vi "输入数据解析.vi"(0 "单个参数补充":dbl, 1 "从板号":dbl=1.0, 2 "主板二维码":string="BNET01", 3 "从板二维码":string="BNET01", 5 "主板引用":refnum<vi>, 7 "从板引用":refnum<vi>, 9 "主板选项":string="三级故障阀值", 11 "枚举":enum16{"主板", "从板"}(ring), 12 "快换":bool caption="快换写入") -> (4 "输出数组":dbl[][](array[numeric]), 6 "数组长度":dbl[](array[numeric]), 8 "循环次数":i32, 10 "命令":u32, 14 "名称":string[](array[string]), 15 "命令序号":u32[](array[numeric]))   [LabVIEW 2013] (continued)
                    n6601 = call "输入分辨率计算-EV05.vi"("1字节?"=FALSE, "数值"=w16862, "分辨率"=0.001) -> ("低字节"=w16864:dbl, "高字节1"=w16865:dbl)  [unwired: 2 in, 5 out]
                  }
                  frame Disabled {
                    w16868 = 255 ("高字节1")
                  }
                }
                n6602 = Build Array(w16861, w16860) -> (w16859:dbl[])
              }
              frame 1 {
                # "电压过低"
                n6603 = disable-structure shown="启用" {
                  disable-tunnel: [w16876 w16879] -> w16872
                  disable-tunnel: [w16875 w16879] -> w16871
                  disable-tunnel: w16869 -> [w16874 _]
                  frame Disabled {
                    n6604 = Unbundle By Name(w16874) -> ("电压过低"=w16873:dbl)
                    n6605 = call "输入分辨率计算-EV05.vi"("1字节?"=FALSE, "数值"=w16873, "分辨率"=0.1) -> ("低字节"=w16875:dbl, "高字节1"=w16876:dbl)  [unwired: 2 in, 5 out]
                  }
                  frame Enabled {
                    w16879 = 255 ("高字节1")
                  }
                }
                n6606 = Build Array(w16872, w16871) -> (w16870:i32[])
              }
              frame 2 {
                # "电压不均衡"
                n6607 = disable-structure shown="启用" {
                  disable-tunnel: [w16887 w16890] -> w16883
                  disable-tunnel: [w16886 w16890] -> w16882
                  disable-tunnel: w16880 -> [w16885 _]
                  frame Disabled {
                    n6608 = Unbundle By Name(w16885) -> ("电压不均衡(V)"=w16884:dbl)
                    n6609 = call "输入分辨率计算-EV05.vi"("1字节?"=FALSE, "数值"=w16884, "分辨率"=0.1) -> ("低字节"=w16886:dbl, "高字节1"=w16887:dbl)  [unwired: 2 in, 5 out]
                  }
                  frame Enabled {
                    w16890 = 255 ("高字节1")
                  }
                }
                n6610 = Build Array(w16883, w16882) -> (w16881:i32[])
              }
              frame 3 {
                # "温度过高"
                n6611 = disable-structure shown="启用" {
                  disable-tunnel: [w16897 255 ("高字节1")] -> w16893
                  disable-tunnel: w16891 -> [w16895 _]
                  frame Disabled {
                    n6612 = Unbundle By Name(w16895) -> ("温度过高"=w16894:dbl)
                    n6613 = call "输入分辨率计算-EV05.vi"("1字节?"=TRUE, "数值"=w16894, "偏移量"=-40.0, "分辨率"=1.0) -> ("高字节1"=w16897:dbl)  [unwired: 1 in, 6 out]
                  }
                  frame Enabled {
                  }
                }
                n6614 = Build Array(w16893) -> (w16892:i32[])
              }
              frame 4 {
                # "温度过低"
                n6615 = disable-structure shown="启用" {
                  disable-tunnel: [w16907 255 ("高字节1")] -> w16903
                  disable-tunnel: w16901 -> [w16905 _]
                  frame Disabled {
                    n6616 = Unbundle By Name(w16905) -> ("温度过低"=w16904:dbl)
                    n6617 = call "输入分辨率计算-EV05.vi"("1字节?"=TRUE, "数值"=w16904, "偏移量"=-40.0, "分辨率"=1.0) -> ("高字节1"=w16907:dbl)  [unwired: 1 in, 6 out]
                  }
                  frame Enabled {
                  }
                }
                n6618 = Build Array(w16903) -> (w16902:i32[])
              }
              frame 5 {
                # "温度不均衡"
                n6619 = disable-structure shown="启用" {
                  disable-tunnel: [w16916 255 ("高字节1")] -> w16913
                  disable-tunnel: w16911 -> [w16915 _]
                  frame Disabled {
                    n6620 = Unbundle By Name(w16915) -> ("温度不均衡"=w16914:dbl)
                    n6621 = call "输入分辨率计算-EV05.vi"("1字节?"=TRUE, "数值"=w16914, "分辨率"=1.0) -> ("高字节1"=w16916:dbl)  [unwired: 2 in, 6 out]
                  }
                  frame Enabled {
                  }
                }
                n6622 = Build Array(w16913) -> (w16912:i32[])
              }
              frame 6 {
                # "SOC过低"
                n6623 = disable-structure shown="启用" {
                  disable-tunnel: w16922 -> [w16939 _]
                  disable-tunnel: [w16925 w16942] -> w16921
                  disable-tunnel: [w16924 w16942] -> w16920
                  frame Disabled {
                    n6624 = Unbundle By Name(w16939) -> ("SOC过低"=w16938:dbl)
                    n6625 = call "输入分辨率计算-EV05.vi"("1字节?"=FALSE, "数值"=w16938, "分辨率"=0.1) -> ("低字节"=w16927:dbl, "高字节1"=w16928:dbl)  [unwired: 2 in, 5 out]
                    n6626 = call "二进制解析-8.6.vi"("索引"=4, "数值"=0) -> ("低位子数组"=w16931:i32[])  [unwired: 3 out]
                    n6627 = call "二进制解析-8.6.vi"("索引"=4, "数值"=w16928) -> ("低位子数组"=w16934:i32[])  [unwired: 3 out]
                    n6628 = call "二进制解析-8.6.vi"("索引"=4, "数值"=w16927) -> ("低位子数组"=w16932:i32[], "高位子数组"=w16933:i32[])  [unwired: 2 out]
                    n6629 = Insert Into Array(array=w16934, new element=w16933) -> (w16936:i32[])  [unwired: 1 in]
                    n6630 = Insert Into Array(array=w16932, new element=w16931) -> (w16930:i32[])  [unwired: 1 in]
                    n6631 = call "数值二进制转十进制-8.6.vi"("子数组"=w16930) -> ("十进制数值"=w16925:i32)  [unwired: 4 out]
                    n6632 = call "数值二进制转十进制-8.6.vi"("子数组"=w16936) -> ("十进制数值"=w16924:i32)  [unwired: 4 out]
                  }
                  frame Enabled {
                    w16942 = 255 ("高字节1")
                  }
                }
                n6633 = Build Array(w16920, w16921) -> (w16923:i32[])
              }
            }
            n6634 = Insert Into Array(array=w16854, new element=w16853) -> (w16855:dbl[])  [unwired: 1 in]
          }
          n6635 = Build Array(w16848) -> (w16847:dbl[][])
        }
        frame "电压过低" {
          n6636 = Unbundle By Name(w16947) -> ("一级故障(从板)"=w16948:refnum<vi>)
          n6637 = property class="Clust (严格)"(reference=w16948) -> ("Value"=w16946:T8)  [unwired: 1 in, 2 out]
          n6638 = for {
            N: 7 -> [_]
            tunnel: w16946 -> [w16958]
            shift-right: [w16957] -> w16950
            shift-left: dbl[] [] -> [w16956]
            i -> [w16959]
            n6639 = case shown="1" w16959 {
              tunnel: w16958 -> [w16960 w16971 w16982 w16993 w17003 w17013 w17024]
              tunnel: [w16961 w16972 w16983 w16994 w17004 w17014 w17025] -> w16955
              frame 0, Default {
                # "电压过高"
                n6640 = disable-structure shown="启用" {
                  disable-tunnel: [w16967 w16970] -> w16963
                  disable-tunnel: [w16966 w16970] -> w16962
                  disable-tunnel: w16960 -> [w16965 _]
                  frame Disabled {
                    n6641 = Unbundle By Name(w16965) -> ("电压过高"=w16964:dbl)
                    n6642 = call "输入分辨率计算-EV05.vi"("1字节?"=FALSE, "数值"=w16964, "分辨率"=0.1) -> ("低字节"=w16966:dbl, "高字节1"=w16967:dbl)  [unwired: 2 in, 5 out]
                  }
                  frame Enabled {
                    w16970 = 255 ("高字节1")
                  }
                }
                n6643 = Build Array(w16963, w16962) -> (w16961:i32[])
              }
              frame 1 {
                # "电压过低"
                n6644 = disable-structure shown="启用" {
                  disable-tunnel: [w16978 w16981] -> w16974
                  disable-tunnel: [w16977 w16981] -> w16973
                  disable-tunnel: w16971 -> [w16976 _]
                  frame Enabled {
                    n6645 = Unbundle By Name(w16976) -> ("电压过低"=w16975:dbl)
                    n6646 = call "输入分辨率计算-EV05.vi"("1字节?"=FALSE, "数值"=w16975, "分辨率"=0.001) -> ("低字节"=w16977:dbl, "高字节1"=w16978:dbl)  [unwired: 2 in, 5 out]
                  }
                  frame Disabled {
                    w16981 = 255 ("高字节1")
                  }
                }
                n6647 = Build Array(w16974, w16973) -> (w16972:dbl[])
              }
              frame 2 {
                # "电压不均衡"
                n6648 = disable-structure shown="启用" {
                  disable-tunnel: [w16989 w16992] -> w16985
                  disable-tunnel: [w16988 w16992] -> w16984
                  disable-tunnel: w16982 -> [w16987 _]
                  frame Disabled {
                    n6649 = Unbundle By Name(w16987) -> ("电压不均衡(V)"=w16986:dbl)
                    n6650 = call "输入分辨率计算-EV05.vi"("1字节?"=FALSE, "数值"=w16986, "分辨率"=0.1) -> ("低字节"=w16988:dbl, "高字节1"=w16989:dbl)  [unwired: 2 in, 5 out]
                  }
                  frame Enabled {
                    w16992 = 255 ("高字节1")
                  }
                }
                n6651 = Build Array(w16985, w16984) -> (w16983:i32[])
              }
              frame 3 {
                # "温度过高"
                n6652 = disable-structure shown="启用" {
                  disable-tunnel: [w16999 255 ("高字节1")] -> w16995
                  disable-tunnel: w16993 -> [w16997 _]
                  frame Disabled {
                    n6653 = Unbundle By Name(w16997) -> ("温度过高"=w16996:dbl)
                    n6654 = call "输入分辨率计算-EV05.vi"("1字节?"=TRUE, "数值"=w16996, "偏移量"=-40.0, "分辨率"=1.0) -> ("高字节1"=w16999:dbl)  [unwired: 1 in, 6 out]
                  }
                  frame Enabled {
                  }
                }
                n6655 = Build Array(w16995) -> (w16994:i32[])
              }
              frame 4 {
                # "温度过低"
                n6656 = disable-structure shown="启用" {
                  disable-tunnel: [w17009 255 ("高字节1")] -> w17005
                  disable-tunnel: w17003 -> [w17007 _]
                  frame Disabled {
                    n6657 = Unbundle By Name(w17007) -> ("温度过低"=w17006:dbl)
                    n6658 = call "输入分辨率计算-EV05.vi"("1字节?"=TRUE, "数值"=w17006, "偏移量"=-40.0, "分辨率"=1.0) -> ("高字节1"=w17009:dbl)  [unwired: 1 in, 6 out]
                  }
                  frame Enabled {
                  }
                }
                n6659 = Build Array(w17005) -> (w17004:i32[])
              }
              frame 5 {
                # "温度不均衡"
                n6660 = disable-structure shown="启用" {
                  disable-tunnel: [w17018 255 ("高字节1")] -> w17015
                  disable-tunnel: w17013 -> [w17017 _]
                  frame Disabled {
                    n6661 = Unbundle By Name(w17017) -> ("温度不均衡"=w17016:dbl)
                    n6662 = call "输入分辨率计算-EV05.vi"("1字节?"=TRUE, "数值"=w17016, "分辨率"=1.0) -> ("高字节1"=w17018:dbl)  [unwired: 2 in, 6 out]
                  }
                  frame Enabled {
                  }
                }
                n6663 = Build Array(w17015) -> (w17014:i32[])
              }
              frame 6 {
                # "SOC过低"
                n6664 = disable-structure shown="启用" {
                  disable-tunnel: w17024 -> [w17041 _]
                  disable-tunnel: [w17027 w17044] -> w17023
                  disable-tunnel: [w17026 w17044] -> w17022
                  frame Disabled {
                    n6665 = Unbundle By Name(w17041) -> ("SOC过低"=w17040:dbl)
                    n6666 = call "输入分辨率计算-EV05.vi"("1字节?"=FALSE, "数值"=w17040, "分辨率"=0.1) -> ("低字节"=w17029:dbl, "高字节1"=w17030:dbl)  [unwired: 2 in, 5 out]
                    n6667 = call "二进制解析-8.6.vi"("索引"=4, "数值"=0) -> ("低位子数组"=w17033:i32[])  [unwired: 3 out]
                    n6668 = call "二进制解析-8.6.vi"("索引"=4, "数值"=w17030) -> ("低位子数组"=w17036:i32[])  [unwired: 3 out]
                    n6669 = call "二进制解析-8.6.vi"("索引"=4, "数值"=w17029) -> ("低位子数组"=w17034:i32[], "高位子数组"=w17035:i32[])  [unwired: 2 out]
                    n6670 = Insert Into Array(array=w17036, new element=w17035) -> (w17038:i32[])  [unwired: 1 in]
                    n6671 = Insert Into Array(array=w17034, new element=w17033) -> (w17032:i32[])  [unwired: 1 in]
                    n6672 = call "数值二进制转十进制-8.6.vi"("子数组"=w17032) -> ("十进制数值"=w17027:i32)  [unwired: 4 out]
                    n6673 = call "数值二进制转十进制-8.6.vi"("子数组"=w17038) -> ("十进制数值"=w17026:i32)  [unwired: 4 out]
                  }
                  frame Enabled {
                    w17044 = 255 ("高字节1")
                  }
                }
                n6674 = Build Array(w17022, w17023) -> (w17025:i32[])
              }
            }
            n6675 = Insert Into Array(array=w16956, new element=w16955) -> (w16957:dbl[])  [unwired: 1 in]
          }
          n6676 = Build Array(w16950) -> (w16949:dbl[][])
        }
        frame "电压过低(2)" {
          n6677 = Unbundle By Name(w17049) -> ("二级故障(从板)"=w17050:refnum<vi>)
          n6678 = property class="Clust (严格)"(reference=w17050) -> ("Value"=w17048:T8)  [unwired: 1 in, 2 out]
          n6679 = for {
            N: 7 -> [_]
            tunnel: w17048 -> [w17060]
            shift-right: [w17059] -> w17052
            shift-left: dbl[] [] -> [w17058]
            i -> [w17061]
            n6680 = case shown="1" w17061 {
              tunnel: w17060 -> [w17062 w17073 w17084 w17095 w17105 w17115 w17126]
              tunnel: [w17063 w17074 w17085 w17096 w17106 w17116 w17127] -> w17057
              frame 0, Default {
                # "电压过高"
                n6681 = disable-structure shown="启用" {
                  disable-tunnel: [w17069 w17072] -> w17065
                  disable-tunnel: [w17068 w17072] -> w17064
                  disable-tunnel: w17062 -> [w17067 _]
                  frame Disabled {
                    n6682 = Unbundle By Name(w17067) -> ("电压过高"=w17066:dbl)
                    n6683 = call "输入分辨率计算-EV05.vi"("1字节?"=FALSE, "数值"=w17066, "分辨率"=0.1) -> ("低字节"=w17068:dbl, "高字节1"=w17069:dbl)  [unwired: 2 in, 5 out]
                  }
                  frame Enabled {
                    w17072 = 255 ("高字节1")
                  }
                }
                n6684 = Build Array(w17065, w17064) -> (w17063:i32[])
              }
              frame 1 {
                # "电压过低"
                n6685 = disable-structure shown="启用" {
                  disable-tunnel: [w17080 w17083] -> w17076
                  disable-tunnel: [w17079 w17083] -> w17075
                  disable-tunnel: w17073 -> [w17078 _]
                  frame Enabled {
                    n6686 = Unbundle By Name(w17078) -> ("电压过低"=w17077:dbl)
                    n6687 = call "输入分辨率计算-EV05.vi"("1字节?"=FALSE, "数值"=w17077, "分辨率"=0.001) -> ("低字节"=w17079:dbl, "高字节1"=w17080:dbl)  [unwired: 2 in, 5 out]
                  }
                  frame Disabled {
                    w17083 = 255 ("高字节1")
                  }
                }
                n6688 = Build Array(w17076, w17075) -> (w17074:dbl[])
              }
              frame 2 {
                # "电压不均衡"
                n6689 = disable-structure shown="启用" {
                  disable-tunnel: [w17091 w17094] -> w17087
                  disable-tunnel: [w17090 w17094] -> w17086
                  disable-tunnel: w17084 -> [w17089 _]
                  frame Disabled {
                    n6690 = Unbundle By Name(w17089) -> ("电压不均衡(V)"=w17088:dbl)
                    n6691 = call "输入分辨率计算-EV05.vi"("1字节?"=FALSE, "数值"=w17088, "分辨率"=0.1) -> ("低字节"=w17090:dbl, "高字节1"=w17091:dbl)  [unwired: 2 in, 5 out]
                  }
                  frame Enabled {
                    w17094 = 255 ("高字节1")
                  }
                }
                n6692 = Build Array(w17087, w17086) -> (w17085:i32[])
              }
              frame 3 {
                # "温度过高"
                n6693 = disable-structure shown="启用" {
                  disable-tunnel: [w17101 255 ("高字节1")] -> w17097
                  disable-tunnel: w17095 -> [w17099 _]
                  frame Disabled {
                    n6694 = Unbundle By Name(w17099) -> ("温度过高"=w17098:dbl)
                    n6695 = call "输入分辨率计算-EV05.vi"("1字节?"=TRUE, "数值"=w17098, "偏移量"=-40.0, "分辨率"=1.0) -> ("高字节1"=w17101:dbl)  [unwired: 1 in, 6 out]
                  }
                  frame Enabled {
                  }
                }
                n6696 = Build Array(w17097) -> (w17096:i32[])
              }
              frame 4 {
                # "温度过低"
                n6697 = disable-structure shown="启用" {
                  disable-tunnel: [w17111 255 ("高字节1")] -> w17107
                  disable-tunnel: w17105 -> [w17109 _]
                  frame Disabled {
                    n6698 = Unbundle By Name(w17109) -> ("温度过低"=w17108:dbl)
                    n6699 = call "输入分辨率计算-EV05.vi"("1字节?"=TRUE, "数值"=w17108, "偏移量"=-40.0, "分辨率"=1.0) -> ("高字节1"=w17111:dbl)  [unwired: 1 in, 6 out]
                  }
                  frame Enabled {
                  }
                }
                n6700 = Build Array(w17107) -> (w17106:i32[])
              }
              frame 5 {
                # "温度不均衡"
                n6701 = disable-structure shown="启用" {
                  disable-tunnel: [w17120 255 ("高字节1")] -> w17117
                  disable-tunnel: w17115 -> [w17119 _]
                  frame Disabled {
                    n6702 = Unbundle By Name(w17119) -> ("温度不均衡"=w17118:dbl)
                    n6703 = call "输入分辨率计算-EV05.vi"("1字节?"=TRUE, "数值"=w17118, "分辨率"=1.0) -> ("高字节1"=w17120:dbl)  [unwired: 2 in, 6 out]
                  }
                  frame Enabled {
                  }
                }
                n6704 = Build Array(w17117) -> (w17116:i32[])
              }
              frame 6 {
                # "SOC过低"
                n6705 = disable-structure shown="启用" {
                  disable-tunnel: w17126 -> [w17143 _]
                  disable-tunnel: [w17129 w17146] -> w17125
                  disable-tunnel: [w17128 w17146] -> w17124
                  frame Disabled {
                    n6706 = Unbundle By Name(w17143) -> ("SOC过低"=w17142:dbl)
                    n6707 = call "输入分辨率计算-EV05.vi"("1字节?"=FALSE, "数值"=w17142, "分辨率"=0.1) -> ("低字节"=w17131:dbl, "高字节1"=w17132:dbl)  [unwired: 2 in, 5 out]
                    n6708 = call "二进制解析-8.6.vi"("索引"=4, "数值"=0) -> ("低位子数组"=w17135:i32[])  [unwired: 3 out]
                    n6709 = call "二进制解析-8.6.vi"("索引"=4, "数值"=w17132) -> ("低位子数组"=w17138:i32[])  [unwired: 3 out]
                    n6710 = call "二进制解析-8.6.vi"("索引"=4, "数值"=w17131) -> ("低位子数组"=w17136:i32[], "高位子数组"=w17137:i32[])  [unwired: 2 out]
                    n6711 = Insert Into Array(array=w17138, new element=w17137) -> (w17140:i32[])  [unwired: 1 in]
                    n6712 = Insert Into Array(array=w17136, new element=w17135) -> (w17134:i32[])  [unwired: 1 in]
                    n6713 = call "数值二进制转十进制-8.6.vi"("子数组"=w17134) -> ("十进制数值"=w17129:i32)  [unwired: 4 out]
                    n6714 = call "数值二进制转十进制-8.6.vi"("子数组"=w17140) -> ("十进制数值"=w17128:i32)  [unwired: 4 out]
                  }
                  frame Enabled {
                    w17146 = 255 ("高字节1")
                  }
                }
                n6715 = Build Array(w17124, w17125) -> (w17127:i32[])
              }
            }
            n6716 = Insert Into Array(array=w17058, new element=w17057) -> (w17059:dbl[])  [unwired: 1 in]
          }
          n6717 = Build Array(w17052) -> (w17051:dbl[][])
        }
        frame "电压过低(3)" {
          n6718 = Unbundle By Name(w17151) -> ("三级故障(从板)"=w17152:refnum<vi>)
          n6719 = property class="Clust (严格)"(reference=w17152) -> ("Value"=w17150:T8)  [unwired: 1 in, 2 out]
          n6720 = for {
            N: 7 -> [_]
            tunnel: w17150 -> [w17162]
            shift-right: [w17161] -> w17154
            shift-left: dbl[] [] -> [w17160]
            i -> [w17163]
            n6721 = case shown="1" w17163 {
              tunnel: w17162 -> [w17164 w17175 w17186 w17197 w17207 w17217 w17228]
              tunnel: [w17165 w17176 w17187 w17198 w17208 w17218 w17229] -> w17159
              frame 0, Default {
                # "电压过高"
                n6722 = disable-structure shown="启用" {
                  disable-tunnel: [w17171 w17174] -> w17167
                  disable-tunnel: [w17170 w17174] -> w17166
                  disable-tunnel: w17164 -> [w17169 _]
                  frame Disabled {
                    n6723 = Unbundle By Name(w17169) -> ("电压过高"=w17168:dbl)
                    n6724 = call "输入分辨率计算-EV05.vi"("1字节?"=FALSE, "数值"=w17168, "分辨率"=0.1) -> ("低字节"=w17170:dbl, "高字节1"=w17171:dbl)  [unwired: 2 in, 5 out]
                  }
                  frame Enabled {
                    w17174 = 255 ("高字节1")
                  }
                }
                n6725 = Build Array(w17167, w17166) -> (w17165:i32[])
              }
              frame 1 {
                # "电压过低"
                n6726 = disable-structure shown="启用" {
                  disable-tunnel: [w17182 w17185] -> w17178
                  disable-tunnel: [w17181 w17185] -> w17177
                  disable-tunnel: w17175 -> [w17180 _]
                  frame Enabled {
                    n6727 = Unbundle By Name(w17180) -> ("电压过低"=w17179:dbl)
                    n6728 = call "输入分辨率计算-EV05.vi"("1字节?"=FALSE, "数值"=w17179, "分辨率"=0.001) -> ("低字节"=w17181:dbl, "高字节1"=w17182:dbl)  [unwired: 2 in, 5 out]
                  }
                  frame Disabled {
                    w17185 = 255 ("高字节1")
                  }
                }
                n6729 = Build Array(w17178, w17177) -> (w17176:dbl[])
              }
              frame 2 {
                # "电压不均衡"
                n6730 = disable-structure shown="启用" {
                  disable-tunnel: [w17193 w17196] -> w17189
                  disable-tunnel: [w17192 w17196] -> w17188
                  disable-tunnel: w17186 -> [w17191 _]
                  frame Disabled {
                    n6731 = Unbundle By Name(w17191) -> ("电压不均衡(V)"=w17190:dbl)
                    n6732 = call "输入分辨率计算-EV05.vi"("1字节?"=FALSE, "数值"=w17190, "分辨率"=0.1) -> ("低字节"=w17192:dbl, "高字节1"=w17193:dbl)  [unwired: 2 in, 5 out]
                  }
                  frame Enabled {
                    w17196 = 255 ("高字节1")
                  }
                }
                n6733 = Build Array(w17189, w17188) -> (w17187:i32[])
              }
              frame 3 {
                # "温度过高"
                n6734 = disable-structure shown="启用" {
                  disable-tunnel: [w17203 255 ("高字节1")] -> w17199
                  disable-tunnel: w17197 -> [w17201 _]
                  frame Disabled {
                    n6735 = Unbundle By Name(w17201) -> ("温度过高"=w17200:dbl)
                    n6736 = call "输入分辨率计算-EV05.vi"("1字节?"=TRUE, "数值"=w17200, "偏移量"=-40.0, "分辨率"=1.0) -> ("高字节1"=w17203:dbl)  [unwired: 1 in, 6 out]
                  }
                  frame Enabled {
                  }
                }
                n6737 = Build Array(w17199) -> (w17198:i32[])
              }
              frame 4 {
                # "温度过低"
                n6738 = disable-structure shown="启用" {
                  disable-tunnel: [w17213 255 ("高字节1")] -> w17209
                  disable-tunnel: w17207 -> [w17211 _]
                  frame Disabled {
                    n6739 = Unbundle By Name(w17211) -> ("温度过低"=w17210:dbl)
                    n6740 = call "输入分辨率计算-EV05.vi"("1字节?"=TRUE, "数值"=w17210, "偏移量"=-40.0, "分辨率"=1.0) -> ("高字节1"=w17213:dbl)  [unwired: 1 in, 6 out]
                  }
                  frame Enabled {
                  }
                }
                n6741 = Build Array(w17209) -> (w17208:i32[])
              }
              frame 5 {
                # "温度不均衡"
                n6742 = disable-structure shown="启用" {
                  disable-tunnel: [w17222 255 ("高字节1")] -> w17219
                  disable-tunnel: w17217 -> [w17221 _]
                  frame Disabled {
                    n6743 = Unbundle By Name(w17221) -> ("温度不均衡"=w17220:dbl)
                    n6744 = call "输入分辨率计算-EV05.vi"("1字节?"=TRUE, "数值"=w17220, "分辨率"=1.0) -> ("高字节1"=w17222:dbl)  [unwired: 2 in, 6 out]
                  }
                  frame Enabled {
                  }
                }
                n6745 = Build Array(w17219) -> (w17218:i32[])
              }
              frame 6 {
                # "SOC过低"
                n6746 = disable-structure shown="启用" {
                  disable-tunnel: w17228 -> [w17245 _]
                  disable-tunnel: [w17231 w17248] -> w17227
                  disable-tunnel: [w17230 w17248] -> w17226
                  frame Disabled {
                    n6747 = Unbundle By Name(w17245) -> ("SOC过低"=w17244:dbl)
                    n6748 = call "输入分辨率计算-EV05.vi"("1字节?"=FALSE, "数值"=w17244, "分辨率"=0.1) -> ("低字节"=w17233:dbl, "高字节1"=w17234:dbl)  [unwired: 2 in, 5 out]
                    n6749 = call "二进制解析-8.6.vi"("索引"=4, "数值"=0) -> ("低位子数组"=w17237:i32[])  [unwired: 3 out]
                    n6750 = call "二进制解析-8.6.vi"("索引"=4, "数值"=w17234) -> ("低位子数组"=w17240:i32[])  [unwired: 3 out]
                    n6751 = call "二进制解析-8.6.vi"("索引"=4, "数值"=w17233) -> ("低位子数组"=w17238:i32[], "高位子数组"=w17239:i32[])  [unwired: 2 out]
                    n6752 = Insert Into Array(array=w17240, new element=w17239) -> (w17242:i32[])  [unwired: 1 in]
                    n6753 = Insert Into Array(array=w17238, new element=w17237) -> (w17236:i32[])  [unwired: 1 in]
                    n6754 = call "数值二进制转十进制-8.6.vi"("子数组"=w17236) -> ("十进制数值"=w17231:i32)  [unwired: 4 out]
                    n6755 = call "数值二进制转十进制-8.6.vi"("子数组"=w17242) -> ("十进制数值"=w17230:i32)  [unwired: 4 out]
                  }
                  frame Enabled {
                    w17248 = 255 ("高字节1")
                  }
                }
                n6756 = Build Array(w17226, w17227) -> (w17229:i32[])
              }
            }
            n6757 = Insert Into Array(array=w17160, new element=w17159) -> (w17161:dbl[])  [unwired: 1 in]
          }
          n6758 = Build Array(w17154) -> (w17153:dbl[][])
        }
        frame "电压不均衡" {
          n6759 = Unbundle By Name(w17253) -> ("一级故障(从板)"=w17254:refnum<vi>)
          n6760 = property class="Clust (严格)"(reference=w17254) -> ("Value"=w17252:T8)  [unwired: 1 in, 2 out]
          n6761 = for {
            N: 7 -> [_]
            tunnel: w17252 -> [w17264]
            shift-right: [w17263] -> w17256
            shift-left: dbl[] [] -> [w17262]
            i -> [w17265]
            n6762 = case shown="3" w17265 {
              tunnel: w17264 -> [w17266 w17277 w17288 w17299 w17309 w17319 w17330]
              tunnel: [w17267 w17278 w17289 w17300 w17310 w17320 w17331] -> w17261
              frame 0, Default {
                # "电压过高"
                n6763 = disable-structure shown="启用" {
                  disable-tunnel: [w17273 w17276] -> w17269
                  disable-tunnel: [w17272 w17276] -> w17268
                  disable-tunnel: w17266 -> [w17271 _]
                  frame Disabled {
                    n6764 = Unbundle By Name(w17271) -> ("电压过高"=w17270:dbl)
                    n6765 = call "输入分辨率计算-EV05.vi"("1字节?"=FALSE, "数值"=w17270, "分辨率"=0.1) -> ("低字节"=w17272:dbl, "高字节1"=w17273:dbl)  [unwired: 2 in, 5 out]
                  }
                  frame Enabled {
                    w17276 = 255 ("高字节1")
                  }
                }
                n6766 = Build Array(w17269, w17268) -> (w17267:i32[])
              }
              frame 1 {
                # "电压过低"
                n6767 = disable-structure shown="启用" {
                  disable-tunnel: [w17284 w17287] -> w17280
                  disable-tunnel: [w17283 w17287] -> w17279
                  disable-tunnel: w17277 -> [w17282 _]
                  frame Disabled {
                    n6768 = Unbundle By Name(w17282) -> ("电压过低"=w17281:dbl)
                    n6769 = call "输入分辨率计算-EV05.vi"("1字节?"=FALSE, "数值"=w17281, "分辨率"=0.1) -> ("低字节"=w17283:dbl, "高字节1"=w17284:dbl)  [unwired: 2 in, 5 out]
                  }
                  frame Enabled {
                    w17287 = 255 ("高字节1")
                  }
                }
                n6770 = Build Array(w17280, w17279) -> (w17278:i32[])
              }
              frame 2 {
                # "电压不均衡"
                n6771 = disable-structure shown="启用" {
                  disable-tunnel: [w17295 w17298] -> w17291
                  disable-tunnel: [w17294 w17298] -> w17290
                  disable-tunnel: w17288 -> [w17293 _]
                  frame Enabled {
                    n6772 = Unbundle By Name(w17293) -> ("电压不均衡(V)"=w17292:dbl)
                    n6773 = call "输入分辨率计算-EV05.vi"("1字节?"=FALSE, "数值"=w17292, "分辨率"=0.001) -> ("低字节"=w17294:dbl, "高字节1"=w17295:dbl)  [unwired: 2 in, 5 out]
                  }
                  frame Disabled {
                    w17298 = 255 ("高字节1")
                  }
                }
                n6774 = Build Array(w17291, w17290) -> (w17289:dbl[])
              }
              frame 3 {
                # "温度过高"
                n6775 = disable-structure shown="启用" {
                  disable-tunnel: [w17305 255 ("高字节1")] -> w17301
                  disable-tunnel: w17299 -> [w17303 _]
                  frame Disabled {
                    n6776 = Unbundle By Name(w17303) -> ("温度过高"=w17302:dbl)
                    n6777 = call "输入分辨率计算-EV05.vi"("1字节?"=TRUE, "数值"=w17302, "偏移量"=-40.0, "分辨率"=1.0) -> ("高字节1"=w17305:dbl)  [unwired: 1 in, 6 out]
                  }
                  frame Enabled {
                  }
                }
                n6778 = Build Array(w17301) -> (w17300:i32[])
              }
              frame 4 {
                # "温度过低"
                n6779 = disable-structure shown="启用" {
                  disable-tunnel: [w17315 255 ("高字节1")] -> w17311
                  disable-tunnel: w17309 -> [w17313 _]
                  frame Disabled {
                    n6780 = Unbundle By Name(w17313) -> ("温度过低"=w17312:dbl)
                    n6781 = call "输入分辨率计算-EV05.vi"("1字节?"=TRUE, "数值"=w17312, "偏移量"=-40.0, "分辨率"=1.0) -> ("高字节1"=w17315:dbl)  [unwired: 1 in, 6 out]
                  }
                  frame Enabled {
                  }
                }
                n6782 = Build Array(w17311) -> (w17310:i32[])
              }
              frame 5 {
                # "温度不均衡"
                n6783 = disable-structure shown="启用" {
                  disable-tunnel: [w17324 255 ("高字节1")] -> w17321
                  disable-tunnel: w17319 -> [w17323 _]
                  frame Disabled {
                    n6784 = Unbundle By Name(w17323) -> ("温度不均衡"=w17322:dbl)
                    n6785 = call "输入分辨率计算-EV05.vi"("1字节?"=TRUE, "数值"=w17322, "分辨率"=1.0) -> ("高字节1"=w17324:dbl)  [unwired: 2 in, 6 out]
                  }
                  frame Enabled {
                  }
                }
                n6786 = Build Array(w17321) -> (w17320:i32[])
              }
              frame 6 {
                # "SOC过低"
                n6787 = disable-structure shown="启用" {
                  disable-tunnel: w17330 -> [w17347 _]
                  disable-tunnel: [w17333 w17350] -> w17329
                  disable-tunnel: [w17332 w17350] -> w17328
                  frame Disabled {
                    n6788 = Unbundle By Name(w17347) -> ("SOC过低"=w17346:dbl)
                    n6789 = call "输入分辨率计算-EV05.vi"("1字节?"=FALSE, "数值"=w17346, "分辨率"=0.1) -> ("低字节"=w17335:dbl, "高字节1"=w17336:dbl)  [unwired: 2 in, 5 out]
                    n6790 = call "二进制解析-8.6.vi"("索引"=4, "数值"=0) -> ("低位子数组"=w17339:i32[])  [unwired: 3 out]
                    n6791 = call "二进制解析-8.6.vi"("索引"=4, "数值"=w17336) -> ("低位子数组"=w17342:i32[])  [unwired: 3 out]
                    n6792 = call "二进制解析-8.6.vi"("索引"=4, "数值"=w17335) -> ("低位子数组"=w17340:i32[], "高位子数组"=w17341:i32[])  [unwired: 2 out]
                    n6793 = Insert Into Array(array=w17342, new element=w17341) -> (w17344:i32[])  [unwired: 1 in]
                    n6794 = Insert Into Array(array=w17340, new element=w17339) -> (w17338:i32[])  [unwired: 1 in]
                    n6795 = call "数值二进制转十进制-8.6.vi"("子数组"=w17338) -> ("十进制数值"=w17333:i32)  [unwired: 4 out]
                    n6796 = call "数值二进制转十进制-8.6.vi"("子数组"=w17344) -> ("十进制数值"=w17332:i32)  [unwired: 4 out]
                  }
                  frame Enabled {
                    w17350 = 255 ("高字节1")
                  }
                }
                n6797 = Build Array(w17328, w17329) -> (w17331:i32[])
              }
            }
            n6798 = Insert Into Array(array=w17262, new element=w17261) -> (w17263:dbl[])  [unwired: 1 in]
          }
          n6799 = Build Array(w17256) -> (w17255:dbl[][])
        }
        frame "电压不均衡(2)" {
          n6800 = Unbundle By Name(w17355) -> ("二级故障(从板)"=w17356:refnum<vi>)
          n6801 = property class="Clust (严格)"(reference=w17356) -> ("Value"=w17354:T8)  [unwired: 1 in, 2 out]
          n6802 = for {
            N: 7 -> [_]
            tunnel: w17354 -> [w17366]
            shift-right: [w17365] -> w17358
            shift-left: dbl[] [] -> [w17364]
            i -> [w17367]
            n6803 = case shown="2" w17367 {
              tunnel: w17366 -> [w17368 w17379 w17390 w17401 w17411 w17421 w17432]
              tunnel: [w17369 w17380 w17391 w17402 w17412 w17422 w17433] -> w17363
              frame 0, Default {
                # "电压过高"
                n6804 = disable-structure shown="启用" {
                  disable-tunnel: [w17375 w17378] -> w17371
                  disable-tunnel: [w17374 w17378] -> w17370
                  disable-tunnel: w17368 -> [w17373 _]
                  frame Disabled {
                    n6805 = Unbundle By Name(w17373) -> ("电压过高"=w17372:dbl)
                    n6806 = call "输入分辨率计算-EV05.vi"("1字节?"=FALSE, "数值"=w17372, "分辨率"=0.1) -> ("低字节"=w17374:dbl, "高字节1"=w17375:dbl)  [unwired: 2 in, 5 out]
                  }
                  frame Enabled {
                    w17378 = 255 ("高字节1")
                  }
                }
                n6807 = Build Array(w17371, w17370) -> (w17369:i32[])
              }
              frame 1 {
                # "电压过低"
                n6808 = disable-structure shown="启用" {
                  disable-tunnel: [w17386 w17389] -> w17382
                  disable-tunnel: [w17385 w17389] -> w17381
                  disable-tunnel: w17379 -> [w17384 _]
                  frame Disabled {
                    n6809 = Unbundle By Name(w17384) -> ("电压过低"=w17383:dbl)
                    n6810 = call "输入分辨率计算-EV05.vi"("1字节?"=FALSE, "数值"=w17383, "分辨率"=0.1) -> ("低字节"=w17385:dbl, "高字节1"=w17386:dbl)  [unwired: 2 in, 5 out]
                  }
                  frame Enabled {
                    w17389 = 255 ("高字节1")
                  }
                }
                n6811 = Build Array(w17382, w17381) -> (w17380:i32[])
              }
              frame 2 {
                # "电压不均衡"
                n6812 = disable-structure shown="启用" {
                  disable-tunnel: [w17397 w17400] -> w17393
                  disable-tunnel: [w17396 w17400] -> w17392
                  disable-tunnel: w17390 -> [w17395 _]
                  frame Enabled {
                    n6813 = Unbundle By Name(w17395) -> ("电压不均衡(V)"=w17394:dbl)
                    n6814 = call "输入分辨率计算-EV05.vi"("1字节?"=FALSE, "数值"=w17394, "分辨率"=0.001) -> ("低字节"=w17396:dbl, "高字节1"=w17397:dbl)  [unwired: 2 in, 5 out]
                  }
                  frame Disabled {
                    w17400 = 255 ("高字节1")
                  }
                }
                n6815 = Build Array(w17393, w17392) -> (w17391:dbl[])
              }
              frame 3 {
                # "温度过高"
                n6816 = disable-structure shown="启用" {
                  disable-tunnel: [w17407 255 ("高字节1")] -> w17403
                  disable-tunnel: w17401 -> [w17405 _]
                  frame Disabled {
                    n6817 = Unbundle By Name(w17405) -> ("温度过高"=w17404:dbl)
                    n6818 = call "输入分辨率计算-EV05.vi"("1字节?"=TRUE, "数值"=w17404, "偏移量"=-40.0, "分辨率"=1.0) -> ("高字节1"=w17407:dbl)  [unwired: 1 in, 6 out]
                  }
                  frame Enabled {
                  }
                }
                n6819 = Build Array(w17403) -> (w17402:i32[])
              }
              frame 4 {
                # "温度过低"
                n6820 = disable-structure shown="启用" {
                  disable-tunnel: [w17417 255 ("高字节1")] -> w17413
                  disable-tunnel: w17411 -> [w17415 _]
                  frame Disabled {
                    n6821 = Unbundle By Name(w17415) -> ("温度过低"=w17414:dbl)
                    n6822 = call "输入分辨率计算-EV05.vi"("1字节?"=TRUE, "数值"=w17414, "偏移量"=-40.0, "分辨率"=1.0) -> ("高字节1"=w17417:dbl)  [unwired: 1 in, 6 out]
                  }
                  frame Enabled {
                  }
                }
                n6823 = Build Array(w17413) -> (w17412:i32[])
              }
              frame 5 {
                # "温度不均衡"
                n6824 = disable-structure shown="启用" {
                  disable-tunnel: [w17426 255 ("高字节1")] -> w17423
                  disable-tunnel: w17421 -> [w17425 _]
                  frame Disabled {
                    n6825 = Unbundle By Name(w17425) -> ("温度不均衡"=w17424:dbl)
                    n6826 = call "输入分辨率计算-EV05.vi"("1字节?"=TRUE, "数值"=w17424, "分辨率"=1.0) -> ("高字节1"=w17426:dbl)  [unwired: 2 in, 6 out]
                  }
                  frame Enabled {
                  }
                }
                n6827 = Build Array(w17423) -> (w17422:i32[])
              }
              frame 6 {
                # "SOC过低"
                n6828 = disable-structure shown="启用" {
                  disable-tunnel: w17432 -> [w17449 _]
                  disable-tunnel: [w17435 w17452] -> w17431
                  disable-tunnel: [w17434 w17452] -> w17430
                  frame Disabled {
                    n6829 = Unbundle By Name(w17449) -> ("SOC过低"=w17448:dbl)
                    n6830 = call "输入分辨率计算-EV05.vi"("1字节?"=FALSE, "数值"=w17448, "分辨率"=0.1) -> ("低字节"=w17437:dbl, "高字节1"=w17438:dbl)  [unwired: 2 in, 5 out]
                    n6831 = call "二进制解析-8.6.vi"("索引"=4, "数值"=0) -> ("低位子数组"=w17441:i32[])  [unwired: 3 out]
                    n6832 = call "二进制解析-8.6.vi"("索引"=4, "数值"=w17438) -> ("低位子数组"=w17444:i32[])  [unwired: 3 out]
                    n6833 = call "二进制解析-8.6.vi"("索引"=4, "数值"=w17437) -> ("低位子数组"=w17442:i32[], "高位子数组"=w17443:i32[])  [unwired: 2 out]
                    n6834 = Insert Into Array(array=w17444, new element=w17443) -> (w17446:i32[])  [unwired: 1 in]
                    n6835 = Insert Into Array(array=w17442, new element=w17441) -> (w17440:i32[])  [unwired: 1 in]
                    n6836 = call "数值二进制转十进制-8.6.vi"("子数组"=w17440) -> ("十进制数值"=w17435:i32)  [unwired: 4 out]
                    n6837 = call "数值二进制转十进制-8.6.vi"("子数组"=w17446) -> ("十进制数值"=w17434:i32)  [unwired: 4 out]
                  }
                  frame Enabled {
                    w17452 = 255 ("高字节1")
                  }
                }
                n6838 = Build Array(w17430, w17431) -> (w17433:i32[])
              }
            }
            n6839 = Insert Into Array(array=w17364, new element=w17363) -> (w17365:dbl[])  [unwired: 1 in]
          }
          n6840 = Build Array(w17358) -> (w17357:dbl[][])
        }
        frame "电压不均衡(3)" {
          n6841 = Unbundle By Name(w17457) -> ("三级故障(从板)"=w17458:refnum<vi>)
          n6842 = property class="Clust (严格)"(reference=w17458) -> ("Value"=w17456:T8)  [unwired: 1 in, 2 out]
          n6843 = for {
            N: 7 -> [_]
            tunnel: w17456 -> [w17468]
            shift-right: [w17467] -> w17460
            shift-left: dbl[] [] -> [w17466]
            i -> [w17469]
            n6844 = case shown="2" w17469 {
              tunnel: w17468 -> [w17470 w17481 w17492 w17503 w17513 w17523 w17534]
              tunnel: [w17471 w17482 w17493 w17504 w17514 w17524 w17535] -> w17465
              frame 0, Default {
                # "电压过高"
                n6845 = disable-structure shown="启用" {
                  disable-tunnel: [w17477 w17480] -> w17473
                  disable-tunnel: [w17476 w17480] -> w17472
                  disable-tunnel: w17470 -> [w17475 _]
                  frame Disabled {
                    n6846 = Unbundle By Name(w17475) -> ("电压过高"=w17474:dbl)
                    n6847 = call "输入分辨率计算-EV05.vi"("1字节?"=FALSE, "数值"=w17474, "分辨率"=0.1) -> ("低字节"=w17476:dbl, "高字节1"=w17477:dbl)  [unwired: 2 in, 5 out]
                  }
                  frame Enabled {
                    w17480 = 255 ("高字节1")
                  }
                }
                n6848 = Build Array(w17473, w17472) -> (w17471:i32[])
              }
              frame 1 {
                # "电压过低"
                n6849 = disable-structure shown="启用" {
                  disable-tunnel: [w17488 w17491] -> w17484
                  disable-tunnel: [w17487 w17491] -> w17483
                  disable-tunnel: w17481 -> [w17486 _]
                  frame Disabled {
                    n6850 = Unbundle By Name(w17486) -> ("电压过低"=w17485:dbl)
                    n6851 = call "输入分辨率计算-EV05.vi"("1字节?"=FALSE, "数值"=w17485, "分辨率"=0.1) -> ("低字节"=w17487:dbl, "高字节1"=w17488:dbl)  [unwired: 2 in, 5 out]
                  }
                  frame Enabled {
                    w17491 = 255 ("高字节1")
                  }
                }
                n6852 = Build Array(w17484, w17483) -> (w17482:i32[])
              }
              frame 2 {
                # "电压不均衡"
                n6853 = disable-structure shown="启用" {
                  disable-tunnel: [w17499 w17502] -> w17495
                  disable-tunnel: [w17498 w17502] -> w17494
                  disable-tunnel: w17492 -> [w17497 _]
                  frame Enabled {
                    n6854 = Unbundle By Name(w17497) -> ("电压不均衡(V)"=w17496:dbl)
                    n6855 = call "输入分辨率计算-EV05.vi"("1字节?"=FALSE, "数值"=w17496, "分辨率"=0.001) -> ("低字节"=w17498:dbl, "高字节1"=w17499:dbl)  [unwired: 2 in, 5 out]
                  }
                  frame Disabled {
                    w17502 = 255 ("高字节1")
                  }
                }
                n6856 = Build Array(w17495, w17494) -> (w17493:dbl[])
              }
              frame 3 {
                # "温度过高"
                n6857 = disable-structure shown="启用" {
                  disable-tunnel: [w17509 255 ("高字节1")] -> w17505
                  disable-tunnel: w17503 -> [w17507 _]
                  frame Disabled {
                    n6858 = Unbundle By Name(w17507) -> ("温度过高"=w17506:dbl)
                    n6859 = call "输入分辨率计算-EV05.vi"("1字节?"=TRUE, "数值"=w17506, "偏移量"=-40.0, "分辨率"=1.0) -> ("高字节1"=w17509:dbl)  [unwired: 1 in, 6 out]
                  }
                  frame Enabled {
                  }
                }
                n6860 = Build Array(w17505) -> (w17504:i32[])
              }
              frame 4 {
                # "温度过低"
                n6861 = disable-structure shown="启用" {
                  disable-tunnel: [w17519 255 ("高字节1")] -> w17515
                  disable-tunnel: w17513 -> [w17517 _]
                  frame Disabled {
                    n6862 = Unbundle By Name(w17517) -> ("温度过低"=w17516:dbl)
                    n6863 = call "输入分辨率计算-EV05.vi"("1字节?"=TRUE, "数值"=w17516, "偏移量"=-40.0, "分辨率"=1.0) -> ("高字节1"=w17519:dbl)  [unwired: 1 in, 6 out]
                  }
                  frame Enabled {
                  }
                }
                n6864 = Build Array(w17515) -> (w17514:i32[])
              }
              frame 5 {
                # "温度不均衡"
                n6865 = disable-structure shown="启用" {
                  disable-tunnel: [w17528 255 ("高字节1")] -> w17525
                  disable-tunnel: w17523 -> [w17527 _]
                  frame Disabled {
                    n6866 = Unbundle By Name(w17527) -> ("温度不均衡"=w17526:dbl)
                    n6867 = call "输入分辨率计算-EV05.vi"("1字节?"=TRUE, "数值"=w17526, "分辨率"=1.0) -> ("高字节1"=w17528:dbl)  [unwired: 2 in, 6 out]
                  }
                  frame Enabled {
                  }
                }
                n6868 = Build Array(w17525) -> (w17524:i32[])
              }
              frame 6 {
                # "SOC过低"
                n6869 = disable-structure shown="启用" {
                  disable-tunnel: w17534 -> [w17551 _]
                  disable-tunnel: [w17537 w17554] -> w17533
                  disable-tunnel: [w17536 w17554] -> w17532
                  frame Disabled {
                    n6870 = Unbundle By Name(w17551) -> ("SOC过低"=w17550:dbl)
                    n6871 = call "输入分辨率计算-EV05.vi"("1字节?"=FALSE, "数值"=w17550, "分辨率"=0.1) -> ("低字节"=w17539:dbl, "高字节1"=w17540:dbl)  [unwired: 2 in, 5 out]
                    n6872 = call "二进制解析-8.6.vi"("索引"=4, "数值"=0) -> ("低位子数组"=w17543:i32[])  [unwired: 3 out]
                    n6873 = call "二进制解析-8.6.vi"("索引"=4, "数值"=w17540) -> ("低位子数组"=w17546:i32[])  [unwired: 3 out]
                    n6874 = call "二进制解析-8.6.vi"("索引"=4, "数值"=w17539) -> ("低位子数组"=w17544:i32[], "高位子数组"=w17545:i32[])  [unwired: 2 out]
                    n6875 = Insert Into Array(array=w17546, new element=w17545) -> (w17548:i32[])  [unwired: 1 in]
                    n6876 = Insert Into Array(array=w17544, new element=w17543) -> (w17542:i32[])  [unwired: 1 in]
                    n6877 = call "数值二进制转十进制-8.6.vi"("子数组"=w17542) -> ("十进制数值"=w17537:i32)  [unwired: 4 out]
                    n6878 = call "数值二进制转十进制-8.6.vi"("子数组"=w17548) -> ("十进制数值"=w17536:i32)  [unwired: 4 out]
                  }
                  frame Enabled {
                    w17554 = 255 ("高字节1")
                  }
                }
                n6879 = Build Array(w17532, w17533) -> (w17535:i32[])
              }
            }
            n6880 = Insert Into Array(array=w17466, new element=w17465) -> (w17467:dbl[])  [unwired: 1 in]
          }
          n6881 = Build Array(w17460) -> (w17459:dbl[][])
        }
        frame "温度过高" {
          n6882 = Unbundle By Name(w17559) -> ("一级故障(从板)"=w17560:refnum<vi>)
          n6883 = property class="Clust (严格)"(reference=w17560) -> ("Value"=w17558:T8)  [unwired: 1 in, 2 out]
          n6884 = for {
            N: 7 -> [_]
            tunnel: w17558 -> [w17570]
            shift-right: [w17569] -> w17562
            shift-left: dbl[] [] -> [w17568]
            i -> [w17571]
            n6885 = case shown="3" w17571 {
              tunnel: w17570 -> [w17572 w17583 w17594 w17605 w17615 w17625 w17636]
              tunnel: [w17573 w17584 w17595 w17606 w17616 w17626 w17637] -> w17567
              frame 0, Default {
                # "电压过高"
                n6886 = disable-structure shown="启用" {
                  disable-tunnel: [w17579 w17582] -> w17575
                  disable-tunnel: [w17578 w17582] -> w17574
                  disable-tunnel: w17572 -> [w17577 _]
                  frame Disabled {
                    n6887 = Unbundle By Name(w17577) -> ("电压过高"=w17576:dbl)
                    n6888 = call "输入分辨率计算-EV05.vi"("1字节?"=FALSE, "数值"=w17576, "分辨率"=0.1) -> ("低字节"=w17578:dbl, "高字节1"=w17579:dbl)  [unwired: 2 in, 5 out]
                  }
                  frame Enabled {
                    w17582 = 255 ("高字节1")
                  }
                }
                n6889 = Build Array(w17575, w17574) -> (w17573:i32[])
              }
              frame 1 {
                # "电压过低"
                n6890 = disable-structure shown="启用" {
                  disable-tunnel: [w17590 w17593] -> w17586
                  disable-tunnel: [w17589 w17593] -> w17585
                  disable-tunnel: w17583 -> [w17588 _]
                  frame Disabled {
                    n6891 = Unbundle By Name(w17588) -> ("电压过低"=w17587:dbl)
                    n6892 = call "输入分辨率计算-EV05.vi"("1字节?"=FALSE, "数值"=w17587, "分辨率"=0.1) -> ("低字节"=w17589:dbl, "高字节1"=w17590:dbl)  [unwired: 2 in, 5 out]
                  }
                  frame Enabled {
                    w17593 = 255 ("高字节1")
                  }
                }
                n6893 = Build Array(w17586, w17585) -> (w17584:i32[])
              }
              frame 2 {
                # "电压不均衡"
                n6894 = disable-structure shown="启用" {
                  disable-tunnel: [w17601 w17604] -> w17597
                  disable-tunnel: [w17600 w17604] -> w17596
                  disable-tunnel: w17594 -> [w17599 _]
                  frame Disabled {
                    n6895 = Unbundle By Name(w17599) -> ("电压不均衡(V)"=w17598:dbl)
                    n6896 = call "输入分辨率计算-EV05.vi"("1字节?"=FALSE, "数值"=w17598, "分辨率"=0.1) -> ("低字节"=w17600:dbl, "高字节1"=w17601:dbl)  [unwired: 2 in, 5 out]
                  }
                  frame Enabled {
                    w17604 = 255 ("高字节1")
                  }
                }
                n6897 = Build Array(w17597, w17596) -> (w17595:i32[])
              }
              frame 3 {
                # "温度过高"
                n6898 = disable-structure shown="启用" {
                  disable-tunnel: [w17611 255 ("高字节1")] -> w17607
                  disable-tunnel: w17605 -> [w17609 _]
                  frame Enabled {
                    n6899 = Unbundle By Name(w17609) -> ("温度过高"=w17608:dbl)
                    n6900 = call "输入分辨率计算-EV05.vi"("1字节?"=TRUE, "数值"=w17608, "偏移量"=-40.0, "分辨率"=1.0) -> ("高字节1"=w17611:dbl)  [unwired: 1 in, 6 out]
                  }
                  frame Disabled {
                  }
                }
                n6901 = Build Array(w17607) -> (w17606:dbl[])
              }
              frame 4 {
                # "温度过低"
                n6902 = disable-structure shown="启用" {
                  disable-tunnel: [w17621 255 ("高字节1")] -> w17617
                  disable-tunnel: w17615 -> [w17619 _]
                  frame Disabled {
                    n6903 = Unbundle By Name(w17619) -> ("温度过低"=w17618:dbl)
                    n6904 = call "输入分辨率计算-EV05.vi"("1字节?"=TRUE, "数值"=w17618, "偏移量"=-40.0, "分辨率"=1.0) -> ("高字节1"=w17621:dbl)  [unwired: 1 in, 6 out]
                  }
                  frame Enabled {
                  }
                }
                n6905 = Build Array(w17617) -> (w17616:i32[])
              }
              frame 5 {
                # "温度不均衡"
                n6906 = disable-structure shown="启用" {
                  disable-tunnel: [w17630 255 ("高字节1")] -> w17627
                  disable-tunnel: w17625 -> [w17629 _]
                  frame Disabled {
                    n6907 = Unbundle By Name(w17629) -> ("温度不均衡"=w17628:dbl)
                    n6908 = call "输入分辨率计算-EV05.vi"("1字节?"=TRUE, "数值"=w17628, "分辨率"=1.0) -> ("高字节1"=w17630:dbl)  [unwired: 2 in, 6 out]
                  }
                  frame Enabled {
                  }
                }
                n6909 = Build Array(w17627) -> (w17626:i32[])
              }
              frame 6 {
                # "SOC过低"
                n6910 = disable-structure shown="启用" {
                  disable-tunnel: w17636 -> [w17653 _]
                  disable-tunnel: [w17639 w17656] -> w17635
                  disable-tunnel: [w17638 w17656] -> w17634
                  frame Disabled {
                    n6911 = Unbundle By Name(w17653) -> ("SOC过低"=w17652:dbl)
                    n6912 = call "输入分辨率计算-EV05.vi"("1字节?"=FALSE, "数值"=w17652, "分辨率"=0.1) -> ("低字节"=w17641:dbl, "高字节1"=w17642:dbl)  [unwired: 2 in, 5 out]
                    n6913 = call "二进制解析-8.6.vi"("索引"=4, "数值"=0) -> ("低位子数组"=w17645:i32[])  [unwired: 3 out]
                    n6914 = call "二进制解析-8.6.vi"("索引"=4, "数值"=w17642) -> ("低位子数组"=w17648:i32[])  [unwired: 3 out]
                    n6915 = call "二进制解析-8.6.vi"("索引"=4, "数值"=w17641) -> ("低位子数组"=w17646:i32[], "高位子数组"=w17647:i32[])  [unwired: 2 out]
                    n6916 = Insert Into Array(array=w17648, new element=w17647) -> (w17650:i32[])  [unwired: 1 in]
                    n6917 = Insert Into Array(array=w17646, new element=w17645) -> (w17644:i32[])  [unwired: 1 in]
                    n6918 = call "数值二进制转十进制-8.6.vi"("子数组"=w17644) -> ("十进制数值"=w17639:i32)  [unwired: 4 out]
                    n6919 = call "数值二进制转十进制-8.6.vi"("子数组"=w17650) -> ("十进制数值"=w17638:i32)  [unwired: 4 out]
                  }
                  frame Enabled {
                    w17656 = 255 ("高字节1")
                  }
                }
                n6920 = Build Array(w17634, w17635) -> (w17637:i32[])
              }
            }
            n6921 = Insert Into Array(array=w17568, new element=w17567) -> (w17569:dbl[])  [unwired: 1 in]
          }
          n6922 = Build Array(w17562) -> (w17561:dbl[][])
        }
        frame "温度过高(2)" {
          n6923 = Unbundle By Name(w17661) -> ("二级故障(从板)"=w17662:refnum<vi>)
          n6924 = property class="Clust (严格)"(reference=w17662) -> ("Value"=w17660:T8)  [unwired: 1 in, 2 out]
          n6925 = for {
            N: 7 -> [_]
            tunnel: w17660 -> [w17672]
            shift-right: [w17671] -> w17664
            shift-left: dbl[] [] -> [w17670]
            i -> [w17673]
            n6926 = case shown="3" w17673 {
              tunnel: w17672 -> [w17674 w17685 w17696 w17707 w17717 w17727 w17738]
              tunnel: [w17675 w17686 w17697 w17708 w17718 w17728 w17739] -> w17669
              frame 0, Default {
                # "电压过高"
                n6927 = disable-structure shown="启用" {
                  disable-tunnel: [w17681 w17684] -> w17677
